vi "Main.vi"() -> ()   [LabVIEW 2013]
uses:
  <vilib>/Utility/error.llb/DialogType.ctl
panel:
  in  "А 2":dbl step=1.0 format="%.1f"
  in  "NeedToSetCurrent 2":bool
  out "В 3":string
  out "А 3":string
  in  "Ручное вкл. 3":bool
  out "Выход 2":bool
  in  "В 2":dbl step=1.0 format="%.3f"
  in  "NeedToSetVoltage 2":bool
  out "message 2":string=" INSTRUCTIONS:\r\rNormal Use:  When using subVIs that incorporate the error in/error out (or error I/O) structure, place this handler where you want to inform the user of an error, typically at the end of the I/O data path, as the last action of the program.  If the error in error? is ERROR, the handler creates a message describing the error and its source.  If the type of dialog = 1 (default), the message is displayed to the user, who can only acknowedge it.  If the type = 2, the user can acknowledge the message or abort execution; aborting a program with active I/O is not recommended.  If the type = 0, no message is displayed; this is used to process the error programmatically, and the error out cluster elements are wired to individual terminals for that reason.  \r\rOther Use:\n\r\nlocal testing.  To test the error code of a subVI or function that does not have the error I/O structure, you can wire its error code and a source string to the local error code and error source inputs.  If error in error? indicates no error and error code is not equal to 0, the local code and source are substituted for the error in values, and error? is set TRUE (ERROR)."
  out "conn src 2":refnum<k5>
  out "conn src":refnum<k5>
  in  "stop":bool
  out "message":string=" INSTRUCTIONS:\r\rNormal Use:  When using subVIs that incorporate the error in/error out (or error I/O) structure, place this handler where you want to inform the user of an error, typically at the end of the I/O data path, as the last action of the program.  If the error in error? is ERROR, the handler creates a message describing the error and its source.  If the type of dialog = 1 (default), the message is displayed to the user, who can only acknowedge it.  If the type = 2, the user can acknowledge the message or abort execution; aborting a program with active I/O is not recommended.  If the type = 0, no message is displayed; this is used to process the error programmatically, and the error out cluster elements are wired to individual terminals for that reason.  \r\rOther Use:\n\r\nlocal testing.  To test the error code of a subVI or function that does not have the error I/O structure, you can wire its error code and a source string to the local error code and error source inputs.  If error in error? indicates no error and error code is not equal to 0, the local code and source are substituted for the error in values, and error? is set TRUE (ERROR)."
  in  "В":dbl step=1.0 format="%.1f"
  in  "А":dbl step=1.0 format="%.1f"
  in  "NeedToSetVoltage":bool
  in  "NeedToSetCurrent":bool
  out "В":string
  out "А":string
  in  "Ручное вкл.":bool
  out "Выход":bool
  # "Линзы дублета HILAC"
  # "Уставка"
  # "Уставка"
  # "F"
  # "D"
  # "Линза F"
  # "Линза D"
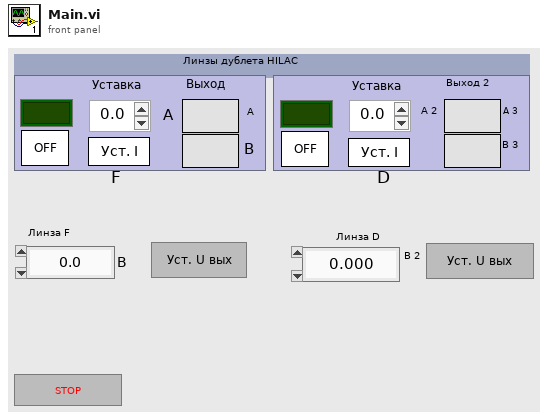
[diagram p1: front panel]
types:
  T1 = typedef "DialogType.ctl" = u16
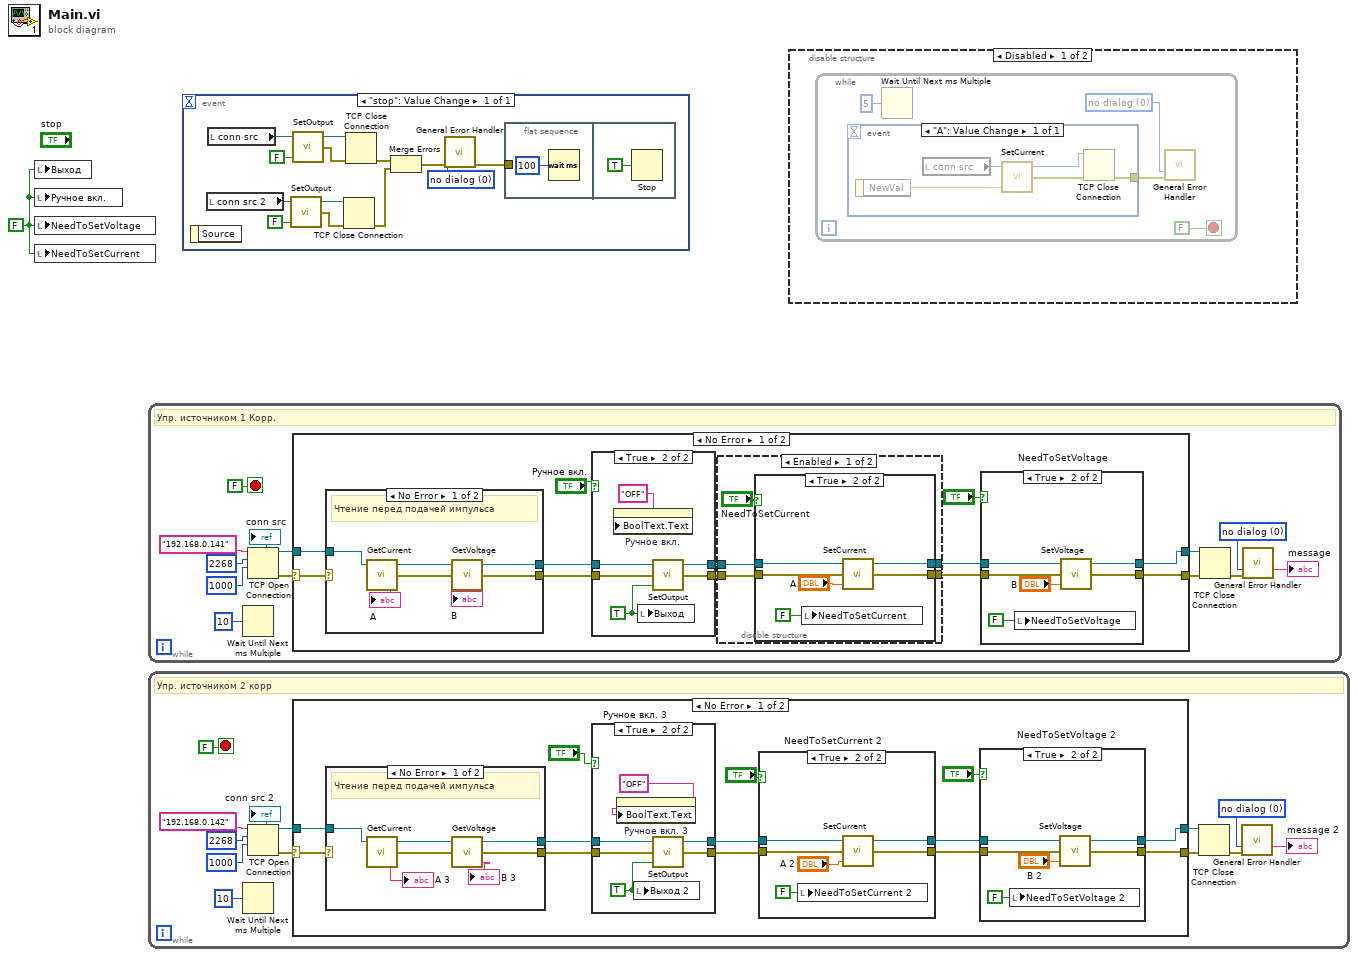
[diagram p0: block diagram]
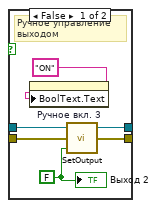
[diagram p3: hidden frame]
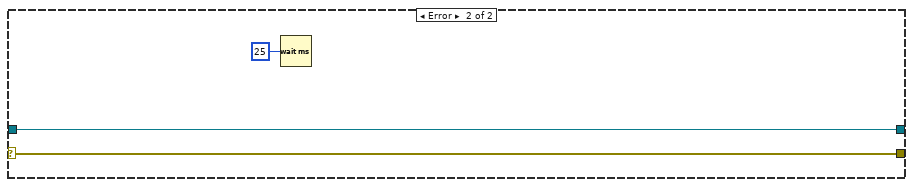
[diagram p7: hidden frame]
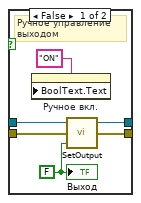
[diagram p10: hidden frame]
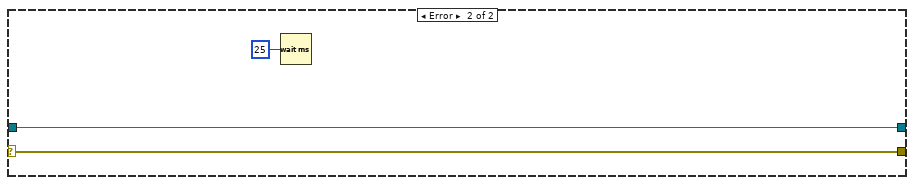
[diagram p13: hidden frame]
diagram:
  w1 = FALSE ("Connect")
  n1 = local write "Выход"(w1) -> ()
  n2 = local write "Ручное вкл."(w1) -> ()
  n3 = local write "NeedToSetVoltage"(w1) -> ()
  n4 = local write "NeedToSetCurrent"(w1) -> ()
  n5 = while {
    stop <- FALSE stop-if-true
    w6 = T1 0 items=["no dialog", "OK message", "continue or stop message", "OK message + warnings", "continue/stop + warnings"] ("type of dialog (OK msg:1)")
    # "Упр. источником 1 Корр."
    n6 = Wait Until Next ms Multiple(millisecond multiple=u32 10 ("milliseconds to wait")) -> ()  [unwired: 1 out]
    n7 = TCP Open Connection(address="192.168.0.141", remote port or service name=u16 2268 ("Port"), timeout ms (60000)=1000) -> (connection ID=w10:refnum<k5>, error out=w11:errorcluster)  [unwired: 1 in, 1 out]
    "conn src" <- w10
    n8 = case shown="No Error" w11 {
      selector: w11 -> [w22 w70]
      tunnel: w10 -> [w21 w71]
      tunnel: [w15 w71] -> w9
      tunnel: [w14 w70] -> w8
      frame No Error {
        n9 = case shown="No Error" w22 {
          selector: w22 -> [_ w60]
          tunnel: w21 -> [w55 w61]
          tunnel: [w54 w60] -> w20
          tunnel: [w53 w61] -> w19
          frame No Error {
            # "Чтение перед подачей импульса"
            n10 = call "GetCurrent.vi"("connection ID"=w55) -> ("Current"=→"А":string, "error out"=w56:errorcluster, "connection ID out"=w58:refnum<k5>)  [unwired: 1 in, 1 out]
            n11 = call "GetVoltage.vi"("error in"=w56, "connection ID"=w58) -> ("Voltage"=→"В":string, "error out"=w54:errorcluster, "connection ID out"=w53:refnum<k5>)  [unwired: 1 out]
          }
          frame Error {
          }
        }
        n12 = case shown="True" "Ручное вкл." {
          tunnel: w20 -> [w46 w52]
          tunnel: w19 -> [w45 w51]
          tunnel: [w43 w50] -> w17
          tunnel: [w42 w49] -> w16
          frame False {
            w44 = FALSE ("State")
            # "Ручное управление выходом"
            n13 = property on="Ручное вкл." class="Bool (strict)"("BoolText.Text"="ON") -> ()  [unwired: 2 in, 2 out]
            n14 = call "SetOutput.vi"("State"=w44, "error in"=w46, "connection ID"=w45) -> ("error out"=w42:errorcluster, "connection ID out"=w43:refnum<k5>)  [unwired: 1 out]
            "Выход" <- w44
          }
          frame True {
            w48 = TRUE ("State")
            n15 = property on="Ручное вкл." class="Bool (strict)"("BoolText.Text"="OFF") -> ()  [unwired: 2 in, 2 out]
            n16 = local write "Выход"(w48) -> ()
            n17 = call "SetOutput.vi"("State"=w48, "error in"=w52, "connection ID"=w51) -> ("error out"=w49:errorcluster, "connection ID out"=w50:refnum<k5>)  [unwired: 1 out]
          }
        }
        n18 = disable-structure shown="Enabled" {
          disable-tunnel: [w30 w40] -> w25
          disable-tunnel: [w28 w39] -> w23
          disable-tunnel: w17 -> [w27 w40]
          disable-tunnel: w16 -> [w26 w39]
          frame Enabled {
            n19 = case shown="True" "NeedToSetCurrent" {
              tunnel: [w32 w37] -> w30
              tunnel: [w31 w35] -> w28
              tunnel: w27 -> [w32 w34]
              tunnel: w26 -> [w31 w33]
              frame False {
              }
              frame True {
                n20 = local write "NeedToSetCurrent"(FALSE ("NeedToSetOutput")) -> ()
                n21 = call "SetCurrent.vi"("Current"="А", "error in"=w33, "connection ID"=w34) -> ("error out"=w35:errorcluster, "connection ID out"=w37:refnum<k5>)  [unwired: 1 out]
              }
            }
          }
          frame Disabled {
          }
        }
        n22 = case shown="True" "NeedToSetVoltage" {
          tunnel: w25 -> [w63 w69]
          tunnel: [w63 w66] -> w15
          tunnel: w23 -> [w62 w65]
          tunnel: [w62 w64] -> w14
          frame False {
          }
          frame True {
            n23 = local write "NeedToSetVoltage"(FALSE ("NeedToSetOutput")) -> ()
            n24 = call "SetVoltage.vi"("Voltage"="В", "error in"=w65, "connection ID"=w69) -> ("error out"=w64:errorcluster, "connection ID out"=w66:refnum<k5>)  [unwired: 1 out]
          }
        }
      }
      frame Error {
        n25 = Wait (ms)(milliseconds to wait=u32 25) -> ()  [unwired: 1 out]
      }
    }
    n26 = TCP Close Connection(connection ID=w9, error in (no error)=w8) -> (error out=w7:errorcluster)  [unwired: 2 out]
    n27 = call <vilib>:"General Error Handler.vi"("type of dialog (OK msg:1)"=w6, "error in (no error)"=w7) -> ("message"=→"message":string)  [unwired: 9 in, 4 out]
  }
  n28 = while {
    stop <- FALSE stop-if-true
    w77 = T1 0 items=["no dialog", "OK message", "continue or stop message", "OK message + warnings", "continue/stop + warnings"] ("type of dialog (OK msg:1)")
    # "Упр. источником 2 корр"
    n29 = Wait Until Next ms Multiple(millisecond multiple=u32 10 ("milliseconds to wait")) -> ()  [unwired: 1 out]
    n30 = TCP Open Connection(address="192.168.0.142", remote port or service name=u16 2268 ("Port"), timeout ms (60000)=1000) -> (connection ID=w81:refnum<k5>, error out=w82:errorcluster)  [unwired: 1 in, 1 out]
    "conn src 2" <- w81
    n31 = case shown="No Error" w82 {
      selector: w82 -> [w94 w135]
      tunnel: w81 -> [w93 w136]
      tunnel: [w88 w136] -> w80
      tunnel: [w87 w135] -> w79
      frame No Error {
        n32 = case shown="No Error" w94 {
          selector: w94 -> [_ w117]
          tunnel: w93 -> [w114 w118]
          tunnel: [w113 w117] -> w92
          tunnel: [w112 w118] -> w91
          frame No Error {
            # "Чтение перед подачей импульса"
            n33 = call "GetCurrent.vi"("connection ID"=w114) -> ("Current"=→"А 3":string, "error out"=w115:errorcluster, "connection ID out"=w116:refnum<k5>)  [unwired: 1 in, 1 out]
            n34 = call "GetVoltage.vi"("error in"=w115, "connection ID"=w116) -> ("Voltage"=→"В 3":string, "error out"=w113:errorcluster, "connection ID out"=w112:refnum<k5>)  [unwired: 1 out]
          }
          frame Error {
          }
        }
        n35 = case shown="True" "Ручное вкл. 3" {
          tunnel: w92 -> [w103 w109]
          tunnel: w91 -> [w102 w108]
          tunnel: [w101 w107] -> w90
          tunnel: [w100 w106] -> w89
          frame False {
            w98 = FALSE ("State")
            # "Ручное управление выходом"
            n36 = property on="Ручное вкл. 3" class="Bool (strict)"("BoolText.Text"="ON") -> ()  [unwired: 2 in, 2 out]
            n37 = call "SetOutput.vi"("State"=w98, "error in"=w103, "connection ID"=w102) -> ("error out"=w100:errorcluster, "connection ID out"=w101:refnum<k5>)  [unwired: 1 out]
            "Выход 2" <- w98
          }
          frame True {
            w105 = TRUE ("State")
            n38 = property on="Ручное вкл. 3" class="Bool (strict)"("BoolText.Text"="OFF") -> ()  [unwired: 2 in, 2 out]
            n39 = local write "Выход 2"(w105) -> ()
            n40 = call "SetOutput.vi"("State"=w105, "error in"=w109, "connection ID"=w108) -> ("error out"=w106:errorcluster, "connection ID out"=w107:refnum<k5>)  [unwired: 1 out]
          }
        }
        n41 = case shown="True" "NeedToSetCurrent 2" {
          tunnel: [w128 w134] -> w97
          tunnel: [w127 w132] -> w95
          tunnel: w90 -> [w128 w131]
          tunnel: w89 -> [w127 w130]
          frame False {
          }
          frame True {
            n42 = local write "NeedToSetCurrent 2"(FALSE ("NeedToSetOutput")) -> ()
            n43 = call "SetCurrent.vi"("Current"="А 2", "error in"=w130, "connection ID"=w131) -> ("error out"=w132:errorcluster, "connection ID out"=w134:refnum<k5>)  [unwired: 1 out]
          }
        }
        n44 = case shown="True" "NeedToSetVoltage 2" {
          tunnel: w97 -> [w120 w126]
          tunnel: [w120 w123] -> w88
          tunnel: w95 -> [w119 w122]
          tunnel: [w119 w121] -> w87
          frame False {
          }
          frame True {
            n45 = local write "NeedToSetVoltage 2"(FALSE ("NeedToSetOutput")) -> ()
            n46 = call "SetVoltage.vi"("Voltage"="В 2", "error in"=w122, "connection ID"=w126) -> ("error out"=w121:errorcluster, "connection ID out"=w123:refnum<k5>)  [unwired: 1 out]
          }
        }
      }
      frame Error {
        n47 = Wait (ms)(milliseconds to wait=u32 25) -> ()  [unwired: 1 out]
      }
    }
    n48 = TCP Close Connection(connection ID=w80, error in (no error)=w79) -> (error out=w78:errorcluster)  [unwired: 2 out]
    n49 = call <vilib>:"General Error Handler.vi"("type of dialog (OK msg:1)"=w77, "error in (no error)"=w78) -> ("message"=→"message 2":string)  [unwired: 9 in, 4 out]
  }
  n50 = event shown="[0] \"stop\": Value Change" {
    selector: _ -> [_]
    dyn-events: _ -> [_]
    timeout: _ -> [_]
    event "stop": Value Change {
      w148 = T1 0 items=["no dialog", "OK message", "continue or stop message", "OK message + warnings", "continue/stop + warnings"] ("type of dialog (OK msg:1)")
      n51 = event-data() -> ()  [unwired: 1 in, 1 out]
      n52 = local read "conn src 2"() -> (w139:refnum<k5>)
      n53 = local read "conn src"() -> (w146:refnum<k5>)
      n54 = call "SetOutput.vi"("State"=FALSE, "connection ID"=w139) -> ("error out"=w141:errorcluster, "connection ID out"=w140:refnum<k5>)  [unwired: 1 in, 1 out]
      n55 = call "SetOutput.vi"("State"=FALSE, "connection ID"=w146) -> ("error out"=w144:errorcluster, "connection ID out"=w145:refnum<k5>)  [unwired: 1 in, 1 out]
      n56 = TCP Close Connection(connection ID=w140, error in (no error)=w141) -> (error out=w138:errorcluster)  [unwired: 1 in, 1 out]
      n57 = TCP Close Connection(connection ID=w145, error in (no error)=w144) -> (error out=w150:errorcluster)  [unwired: 1 in, 1 out]
      n58 = Merge Errors(w150, w138) -> (w149:errorcluster)
      n59 = call <vilib>:"General Error Handler.vi"("type of dialog (OK msg:1)"=w148, "error in (no error)"=w149) -> ("error out"=w147:errorcluster)  [unwired: 9 in, 4 out]
      n60 = flat-sequence {
        tunnel: w147 -> [_]
        frame #0 {
          n61 = Wait (ms)(milliseconds to wait=u32 100) -> ()  [unwired: 1 out]
        }
        frame #1 {
          n62 = Stop(stop? (T)=TRUE) -> ()
        }
      }
    }
  }
  n63 = disable-structure shown="Disabled" {
    frame Disabled {
      n64 = while {
        stop <- FALSE stop-if-true
        w156 = T1 0 items=["no dialog", "OK message", "continue or stop message", "OK message + warnings", "continue/stop + warnings"] ("type of dialog (OK msg:1)")
        n65 = event shown="[0] \"А\": Value Change" {
          selector: _ -> [_]
          dyn-events: _ -> [_]
          timeout: _ -> [_]
          tunnel: [w157] -> w155
          event "А": Value Change {
            n66 = event-data() -> ("NewVal"=w161:dbl)  [unwired: 1 in]
            n67 = local read "conn src"() -> (w160:refnum<k5>)
            n68 = call "SetCurrent.vi"("Current"=w161, "connection ID"=w160) -> ("error out"=w158:errorcluster, "connection ID out"=w159:refnum<k5>)  [unwired: 1 in, 1 out]
            n69 = TCP Close Connection(connection ID=w159, error in (no error)=w158) -> (error out=w157:errorcluster)  [unwired: 2 out]
          }
        }
        n70 = Wait Until Next ms Multiple(millisecond multiple=u32 5) -> ()  [unwired: 1 out]
        n71 = call <vilib>:"General Error Handler.vi"("type of dialog (OK msg:1)"=w156, "error in (no error)"=w155) -> ()  [unwired: 9 in, 5 out]
      }
    }
    frame Enabled {
    }
  }
